vi "Abstract MVA Application Template.vi"   [LabVIEW 2017]
uses:
  Framework/IModel/IModel/IModel.lvclass
  C:/Git/mva-framework/Source/Framework/IObserver/IObserver/IObserver.lvclass
  Framework/IViewable/IViewable/IViewable.lvclass
  Framework/IViewModel/IViewModel/IViewModel.lvclass
  C:/Git/mva-framework/Source/Framework/IViewManager/IViewManager/IViewManager.lvclass
  C:/Program Files (x86)/National Instruments/LabVIEW 2017/vi.lib/ActorFramework/Actor/Actor.lvclass
  Framework/Mediator/Mediator/Mediator.lvclass
  C:/Git/mva-framework/Source/Framework/IMediator/IMediator/IMediator.lvclass
  Framework/Mediator/MediatorBusMonitor/MediatorBusMonitor.lvclass
  C:/Git/mva-framework/Source/Framework/IMediator/IMediatorBusMonitor/IMediatorBusMonitor.lvclass
  <vilib>/ActorFramework/Message Enqueuer/Message Priority.ctl
  Framework/IViewable/IViewable/View Position Enum.ctl
  Framework/IObserver/IObserver/IObserver.lvclass/IObserver.ctl
  Framework/IMediator/IMediator/IMediator.lvclass/IMediator.ctl
  Framework/IViewModel/IViewModel/IViewModel.lvclass/IViewModel.ctl
  Framework/IViewManager/IViewManager Messages/Launch Nested Views Msg/Launch Nested Views Msg.lvclass/Launch Nested Views Msg.ctl
  Framework/IViewManager/IViewManager/IViewManager.lvclass/IViewManager.ctl
  Framework/IViewable/IViewable Messages/Open Front Panel Msg/Open Front Panel Msg.lvclass/Open Front Panel Msg.ctl
  <vilib>/ActorFramework/Message Enqueuer/Message Enqueuer.lvclass/Message Enqueuer.ctl
  5c4f144a-bf04-4631-b5b9-56dc2cdea438.vi
  Framework/IObserver/IObserver/Configure Observer Logging.vi
  Framework/IViewModel/IViewModel/Write Startup Model-View Configuration.vi
  Framework/IMediator/IMediator/Configure Mediator.vi
  <vilib>/ActorFramework/Message Enqueuer/Enqueue.vi
  Framework/IViewManager/IViewManager Messages/Launch Nested Views Msg/Pack Launch Nested Views Msg.vi
  Framework/IViewManager/IViewManager/Write Startup Launch Nested Views Msg.vi
  Framework/IViewable/IViewable Messages/Open Front Panel Msg/Open Front Panel Msg.lvclass
  C:/Program Files (x86)/National Instruments/LabVIEW 2017/vi.lib/ActorFramework/Message/Message.lvclass
  <vilib>/ActorFramework/Message Priority Queue/Priority Enqueue.vi
  gpm_packages/@cs/event-logger/Source/Composed Log/LoggerReference/LoggerReference.lvclass
  Framework/IViewable/IApplicationStyle/IApplicationStyle.lvclass
  Framework/IViewManager/IViewManager Messages/Launch Nested Views Msg/Launch Nested Views Msg.lvclass
  <vilib>/ActorFramework/Actor/Actor.lvclass
  <vilib>/ActorFramework/Message Enqueuer/Message Enqueuer.lvclass
  EventSinkConfigurations/EventSinkConfigurations.lvlib
panel:
  # "This example launches a simple abstract MVA application.\nReplace IModel with your Root Model or dependency-injected Model hierarchy.\nReplace IViewable with your Viewable or nested hierarchy of Viewables and ViewManagers\nReplace IViewModel with your concrete ViewModel that requests Model activity driven by user inputs\nMediator is already concrete--only replace it if you write your own Mediator"
types:
  T1 = typedef "IViewable.lvlib/IViewable.lvclass/View Position Enum.ctl" = enum16{"Centered", "Maximized", "Minimized", "Custom", "Unchanged"}
  T2 = typedef "Actor Framework.lvlib/Message Enqueuer.lvclass/Message Priority.ctl" = enum16{"Low", "Normal", "High"}
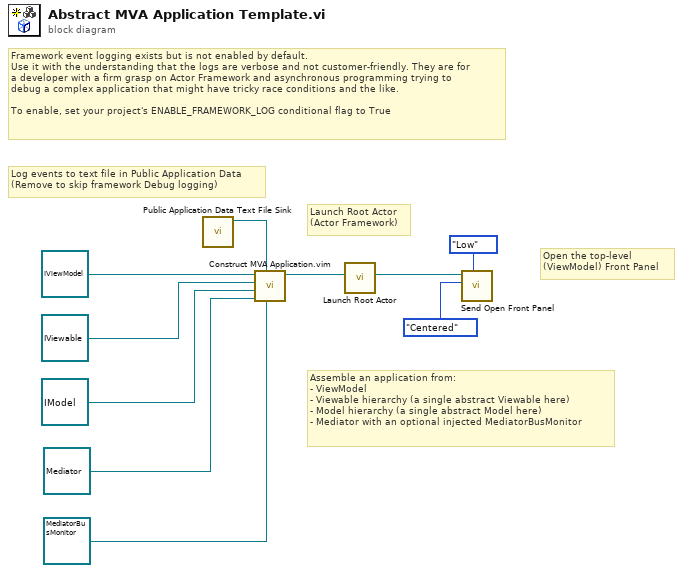
[diagram p0: block diagram]
diagram:
  # "Framework event logging exists but is not enabled by default.\nUse it with the understanding that the logs are verbose and not customer-friendly. They are for\na developer with a firm grasp on Actor Framework and asynchronous programming trying to\ndebug a complex application that might have tricky race conditions and the like.\n\nTo enable, set your project's ENABLE_FRAMEWORK_LOG conditional flag to True"
  # "Log events to text file in Public Application Data\n(Remove to skip framework Debug logging)"
  # "Open the top-level\n(ViewModel) Front Panel"
  # "Launch Root Actor\n(Actor Framework)"
  # "Assemble an application from:\n- ViewModel\n- Viewable hierarchy (a single abstract Viewable here)\n- Model hierarchy (a single abstract Model here)\n- Mediator with an optional injected MediatorBusMonitor"
  n1 = call "Public Application Data Text File Sink.vi"() -> ("Text File Sink"=w1:refnum<class "Text File Sink.lvclass">)  [unwired: 11 in]
  n2 = call "Construct MVA Application.vim"("MediatorBusMonitor Type"=refnum<class "MediatorBusMonitor.lvclass"> refnum ("Mediator.lvlib:MediatorBusMonitor.lvclass"), "Event Log Sink(s)"=w1, "Mediator Type"=refnum<class "Mediator.lvclass"> refnum ("Mediator.lvlib:Mediator.lvclass"), "Model Type"=refnum<class "IModel.lvclass"> refnum ("IModel.lvlib:IModel.lvclass"), "Startup View Configuration"=refnum<class "IViewable.lvclass"> refnum ("IViewable.lvlib:IViewable.lvclass"), "IViewModel In"=refnum<class "IViewModel.lvclass"> refnum ("IViewModel.lvlib:IViewModel.lvclass")) -> ("IViewModel Out"=w7:refnum<class "IViewModel.lvclass">)  [unwired: 5 in]
  n3 = call <vilib>:"Launch Root Actor.vi"("Actor"=w7) -> ("Actor's Enqueuer"=w6:refnum<class "Message Enqueuer.lvclass">)  [unwired: 9 in, 1 out]
  n4 = call "Send Open Front Panel.vi"("Message Priority (Normal)"=Message_Priority."Low", "Position"=View_Position_Enum."Centered", "Message Enqueuer"=w6) -> ()  [unwired: 7 in, 2 out]
